vi "Report Creator.vi"(8 "date":string="total", 9 "Affiliate Weekly Path":path=path "C:/Dropbox/The_Student_Book_Project_LLC/Reports/affiliate.csv", 11 "Merch Weekly Path":path=path "C:/Dropbox/The_Student_Book_Project_LLC/Reports/Merchandise.csv") -> ()   [LabVIEW 2010]
uses:
  <vilib>/Utility/file.llb/Read From Spreadsheet File (string).vi
  <vilib>/Utility/file.llb/Write To Spreadsheet File (string).vi
  <vilib>/Analysis/NI_AALBase.lvlib
panel:
  out "Total Good Matches":string[][](array[string])
  out "Muliples Decided as Single":string[][](array[string])
  out "Levianthing 5":u8
  out "Levianthing 4":u8
  out "Levianthing 3":u8
  out "Levianthin 2":u8
  out "Affiliate Row # 5":i32
  out "Affiliate Row # 4":i32
  out "Affiliate Row # 3":i32
  out "Affiliate Row # 2":i32
  out "size(s)":i32
  out "Single Good Array":string[](array[string])
  out "Good Single Match Books per Org":string[][](array[string])
  out "Aggregated Good Multiple Match Books per Org":string[][](array[string])
  out "number of good, multiple matches":dbl
  out "Book Identifier":string
  out "Extension":string
  in  "Cutoff for Levianthing":u8=10
  out "Match Link 5":string
  out "Match Link 4":string
  out "Match Link 3":string
  out "Match Link 2":string
  out "Single Match Link":string
  out "Book Commission":string
  out "Book Revenue":string
  out "Book Name Merchandise":string
  out "Merchandise Data":string[][](array[string])
  out "Affiliate Row #":i32
  out "Merchandise row #":i32
  out "Single Match":bool
  out "Histogram Graph 2":T1(graph)
  out "number of good, single matches":dbl
  out "number not single and greater than 10":dbl
  out "number of bad matches":dbl
  out "number of good matches":dbl
  out "number of single matches":dbl
  out "number of multiple matches":dbl
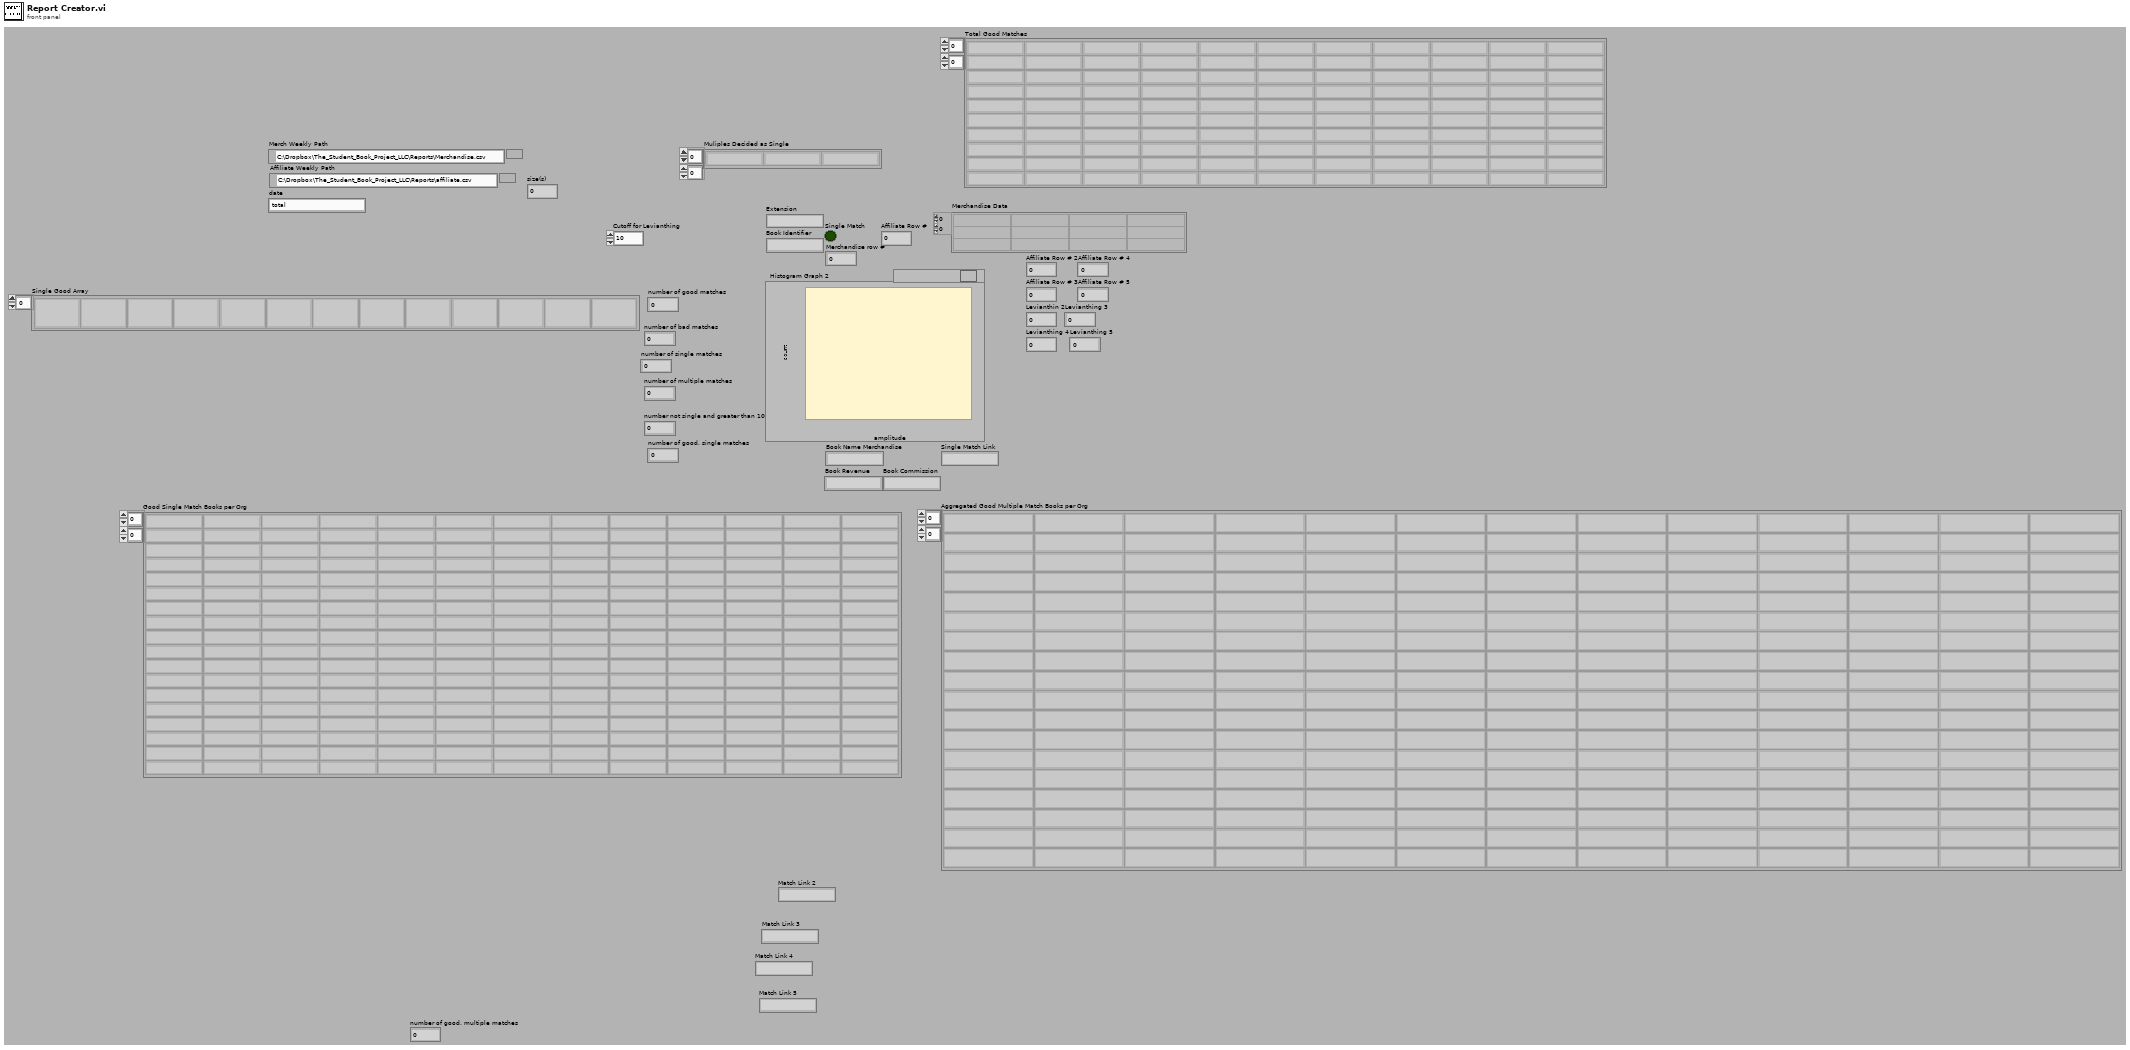
[diagram p1: front panel]
types:
  T1 = cluster{"X Values":dbl[], "Histogram: h(x)":i32[]}
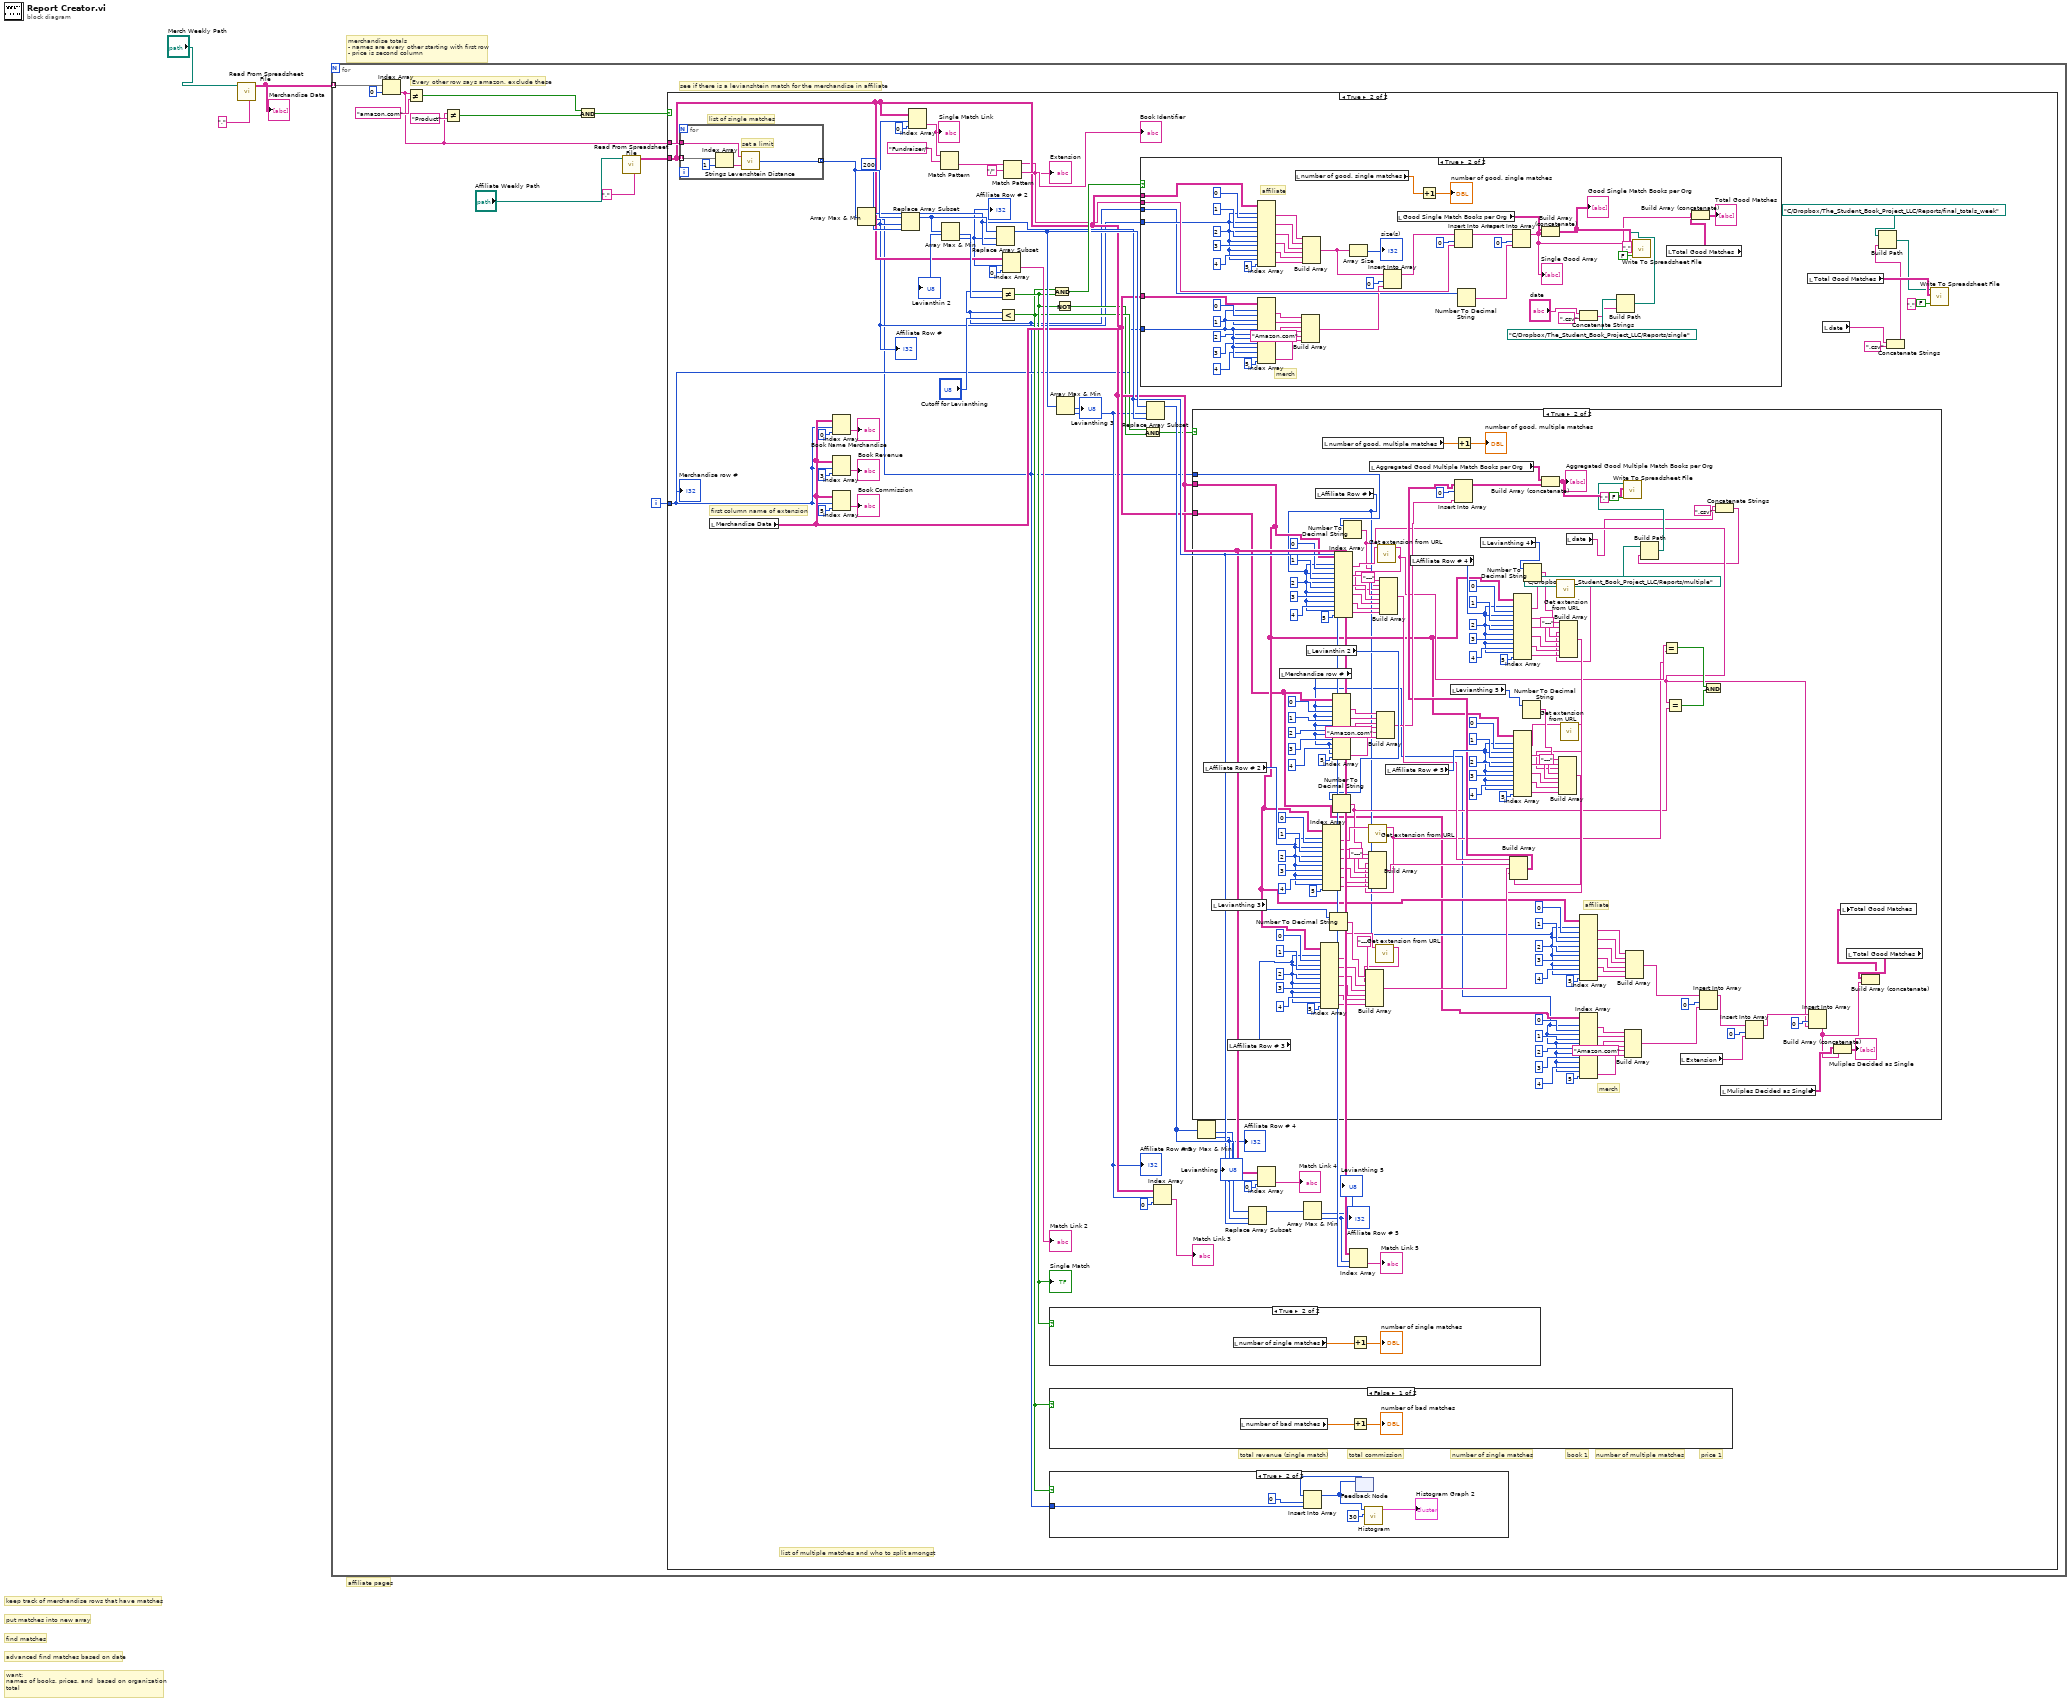
[diagram p0: block diagram]
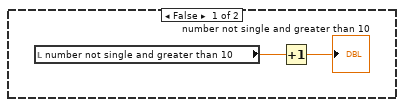
[diagram p5: hidden frame]
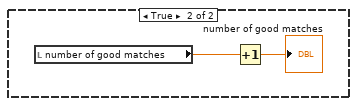
[diagram p6: hidden frame]
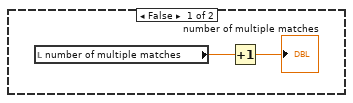
[diagram p7: hidden frame]
diagram:
  # "want:\nnames of books, prices, and  based on organization\ntotal"
  # "put matches into new array"
  # "keep track of merchandise rows that have matches"
  # "advanced find matches based on date"
  # "find matches"
  # "affiliate pages"
  # "merchandise totals\n- names are every other starting with first row\n- price is second column"
  n1 = call-poly <vilib>:"Read From Spreadsheet File.vi"("delimiter (\\t)"="," ("delimiter (\\t)"), "file path (dialog if empty)"="Merch Weekly Path") -> ("all rows"=w3:string[][])  [unwired: 5 in, 4 out]
  "Merchandise Data" <- w3
  n2 = for {
    tunnel: w3 -> [w10] mode=indexing
    i -> [w7]
    # "Every other row says amazon, exclude these"
    # "see if there is a levianshtein match for the merchandise in affiliate"
    n3 = Index Array(array=w10, index=0) -> (element=w9:string)
    n4 = Not Equal?(x=w9, y="amazon.com") -> (x != y?=w12:bool)
    n5 = Not Equal?(x=w9, y="Product") -> (x != y?=w11:bool)
    n6 = And(x=w12, y=w11) -> (x .and. y?=w5:bool)
    n7 = call-poly <vilib>:"Read From Spreadsheet File.vi"("delimiter (\\t)"="," ("delimiter (\\t)"), "file path (dialog if empty)"="Affiliate Weekly Path") -> ("all rows"=w6:string[][])  [unwired: 5 in, 4 out]
    n8 = case shown="True" w5 {
      tunnel: w9 -> [_ w69]
      tunnel: w6 -> [_ w39]
      tunnel: w7 -> [_ w33]
      frame False {
      }
      frame True {
        w46 = u8 200 ("new element/subarray")
        # "list of multiple matches and who to split amongst"
        # "list of single matches"
        # "total revenue (single match)"
        # "price 1"
        # "book 1"
        # "number of multiple matches"
        # "number of single matches"
        # "total commission"
        # "first column name of extension"
        n9 = for {
          tunnel: w69 -> [w302]
          tunnel: w39 -> [w301] mode=indexing
          tunnel: [w298] -> w68 mode=indexing
          # "set a limit"
          n10 = Index Array(array=w301, index=1) -> (element=w299:string)
          n11 = call "Strings Levenshtein Distance.vi"("String 2"=w299, "String 1"=w302) -> ("distance"=w298:u8)
        }
        n12 = local read "Merchandise Data"() -> (w40:string[][])
        n13 = Index Array(array=w40, index (row)=w33, index (col)=0 ("disabled index (col)")) -> (element=→"Book Name Merchandise":string)
        n14 = Index Array(array=w40, index (row)=w33, index (col)=3 ("disabled index (col)")) -> (element=→"Book Revenue":string)
        n15 = Index Array(array=w40, index (row)=w33, index (col)=5 ("disabled index (col)")) -> (element=→"Book Commission":string)
        n16 = Array Max & Min(array=w68) -> (min value=w27:u8, min index (indices)=w32:i32)  [unwired: 2 out]
        "Affiliate Row #" <- w32
        n17 = Replace Array Subset(array=w68, new element=w46, index=w32) -> (w66:u8[])
        n18 = Index Array(array=w39, index (row)=w32, index (col)=0 ("disabled index (col)")) -> (element=w45:string)
        "Single Match Link" <- w45
        n19 = Match Pattern(string=w45, regular expression="Fundraiser/") -> (after substring=w43:string)  [unwired: 1 in, 3 out]
        n20 = Array Max & Min(array=w66) -> (min value=w67:u8, min index (indices)=w31:i32)  [unwired: 2 out]
        "Affiliate Row # 2" <- w31
        "Levianthin 2" <- w67
        n21 = Replace Array Subset(array=w66, new element=w46, index=w31) -> (w49:u8[])
        n22 = Not Equal?(x=w27, y=w67) -> (x != y?=w38:bool)
        "Single Match" <- w38
        n23 = Less?(x=w27, y="Cutoff for Levianthing") -> (x < y?=w37:bool)
        n24 = Index Array(array=w39, index (row)=w31, index (col)=0 ("disabled index (col)")) -> (element=→"Match Link 2":string)
        n25 = Match Pattern(string=w43, regular expression="/") -> (before substring=w34:string, after substring=→"Book Identifier":string)  [unwired: 1 in, 2 out]
        "Extension" <- w34
        n26 = case shown="True" w38 {
          frame False {
            n27 = local read "number of multiple matches"() -> (w294:dbl)
            n28 = Increment(x=w294) -> (x+1=→"number of multiple matches":dbl)
          }
          frame True {
            n29 = local read "number of single matches"() -> (w296:dbl)
            n30 = Increment(x=w296) -> (x+1=→"number of single matches":dbl)
          }
        }
        n31 = case shown="False" w37 {
          frame False {
            n32 = local read "number of bad matches"() -> (w290:dbl)
            n33 = Increment(x=w290) -> (x+1=→"number of bad matches":dbl)
          }
          frame True {
            n34 = local read "number of good matches"() -> (w292:dbl)
            n35 = Increment(x=w292) -> (x+1=→"number of good matches":dbl)
          }
        }
        n36 = case shown="True" w37 {
          tunnel: w27 -> [_ w234]
          frame False {
          }
          frame True {
            n37 = feedback #1() -> (w230:u8[])  [unwired: 1 in]
            n38 = Insert Into Array(array=w230, index=0, new element=w234) -> (w229:u8[])
            n39 = feedback-in #1(w229) -> ()
            n40 = call <vilib>:"Histogram.vi"("intervals"=30, "X"=w229) -> ("Histogram Graph"=→"Histogram Graph 2":T1)  [unwired: 6 in, 3 out]
          }
        }
        n41 = And(x=w37, y=w38) -> (x .and. y?=w65:bool)
        n42 = Not(x=w38) -> (.not. x?=w36:bool)
        n43 = Array Max & Min(array=w49) -> (min value=→"Levianthing 3":u8, min index (indices)=w30:i32)  [unwired: 2 out]
        "Affiliate Row # 3" <- w30
        n44 = case shown="True" w65 {
          tunnel: w40 -> [_ w287]
          tunnel: w39 -> [_ w267]
          tunnel: w34 -> [_ w284]
          tunnel: w33 -> [_ w279]
          tunnel: w32 -> [_ w259]
          tunnel: w27 -> [_ w252]
          frame False {
            n45 = local read "number not single and greater than 10"() -> (w235:dbl)
            n46 = Increment(x=w235) -> (x+1=→"number not single and greater than 10":dbl)
          }
          frame True {
            # "merch"
            # "affiliate"
            n47 = Index Array(array=w267, index (row) #1=w259, index (col) #1=0 ("disabled index (col)"), index (row) #2=w259, index (col) #2=1 ("disabled index (col)"), index (row) #3=w259, index (col) #3=2 ("disabled index (col)"), index (row) #4=w259, index (col) #4=3 ("disabled index (col)"), index (row) #5=w259, index (col) #5=4 ("disabled index (col)"), index (row) #6=w259, index (col) #6=5 ("disabled index (col)")) -> (element #1=w266:string, element #2=w260:string, element #3=w258:string, element #4=w257:string, element #5=w256:string, element #6=w255:string)
            n48 = Index Array(array=w287, index (row) #1=w279, index (col) #1=0 ("disabled index (col)"), index (row) #2=w279, index (col) #2=1 ("disabled index (col)"), index (row) #3=w279, index (col) #3=2 ("disabled index (col)"), index (row) #4=w279, index (col) #4=3 ("disabled index (col)"), index (row) #5=w279, index (col) #5=4 ("disabled index (col)"), index (row) #6=w279, index (col) #6=5 ("disabled index (col)")) -> (element #1=w281:string, element #2=w264:string, element #3=w263:string, element #4=w262:string, element #6=w261:string)  [unwired: 1 out]
            n49 = local read "number of good, single matches"() -> (w288:dbl)
            n50 = Build Array(w281, w264, w263, w262, "Amazon.com" ("element"), w261) -> (w280:string[])
            n51 = Build Array(w266, w260, w258, w257, w256, w255) -> (w265:string[])
            n52 = Array Size(array=w265) -> (size(s)=→"size(s)":i32)
            n53 = Insert Into Array(array=w265, index=0, new element=w280) -> (w250:string[])
            n54 = local read "Good Single Match Books per Org"() -> (w254:string[][])
            n55 = Increment(x=w288) -> (x+1=→"number of good, single matches":dbl)
            n56 = Insert Into Array(array=w250, index=0, new element=w284) -> (w249:string[])
            n57 = Number To Decimal String(number=w252) -> (decimal integer string=w251:string)  [unwired: 1 in]
            n58 = Insert Into Array(array=w249, index=0, new element=w251) -> (w243:string[])
            "Single Good Array" <- w243
            n59 = Build Array (concatenate)(w254, w243) -> (w248:string[][])
            "Good Single Match Books per Org" <- w248
            n60 = Concatenate Strings("date", ".csv" ("string")) -> (w238:string)
            n61 = Build Path(base path=path "C:/Dropbox/The_Student_Book_Project_LLC/Reports/single" ("file path (dialog if empty)"), name or relative path=w238) -> (appended path=w244:path)
            n62 = call-poly <vilib>:"Write To Spreadsheet File.vi"("delimiter (\\t)"="," ("delimiter (\\t)"), "append to file? (new file:F)"=FALSE, "2D data"=w248, "file path (dialog if empty)"=w244) -> ()  [unwired: 4 in, 1 out]
            n63 = local read "Total Good Matches"() -> (w241:string[][])
            n64 = Build Array (concatenate)(w241, w243) -> (→"Total Good Matches":string[][])
          }
        }
        n65 = And(x=w37, y=w36) -> (x .and. y?=w35:bool)
        n66 = Replace Array Subset(array=w49, new element=w46, index=w30) -> (w48:u8[])
        n67 = Index Array(array=w39, index (row)=w30, index (col)=0 ("disabled index (col)")) -> (element=→"Match Link 3":string)
        n68 = case shown="True" w35 {
          tunnel: w40 -> [_ w90]
          tunnel: w39 -> [_ w92]
          tunnel: w27 -> [_ w202]
          frame False {
          }
          frame True {
            # "merch"
            # "affiliate"
            n69 = local read "Affiliate Row # 2"() -> (w149:i32)
            n70 = local read "Levianthing 3"() -> (w144:u8)
            n71 = local read "Affiliate Row # 3"() -> (w148:i32)
            n72 = local read "Merchandise row #"() -> (w89:i32)
            n73 = local read "Levianthin 2"() -> (w145:u8)
            n74 = local read "Affiliate Row #"() -> (w91:i32)
            n75 = Index Array(array=w92, index (row) #1=w148, index (col) #1=0 ("disabled index (col)"), index (row) #2=w148, index (col) #2=1 ("disabled index (col)"), index (row) #3=w148, index (col) #3=2 ("disabled index (col)"), index (row) #4=w148, index (col) #4=3 ("disabled index (col)"), index (row) #5=w148, index (col) #5=4 ("disabled index (col)"), index (row) #6=w148, index (col) #6=5 ("disabled index (col)")) -> (element #1=w132:string, element #2=w182:string, element #3=w181:string, element #4=w180:string, element #5=w179:string, element #6=w178:string)
            n76 = local read "number of good, multiple matches"() -> (w227:dbl)
            n77 = Index Array(array=w92, index (row) #1=w149, index (col) #1=0 ("disabled index (col)"), index (row) #2=w149, index (col) #2=1 ("disabled index (col)"), index (row) #3=w149, index (col) #3=2 ("disabled index (col)"), index (row) #4=w149, index (col) #4=3 ("disabled index (col)"), index (row) #5=w149, index (col) #5=4 ("disabled index (col)"), index (row) #6=w149, index (col) #6=5 ("disabled index (col)")) -> (element #1=w133:string, element #2=w194:string, element #3=w193:string, element #4=w192:string, element #5=w191:string, element #6=w190:string)
            n78 = Number To Decimal String(number=w144) -> (decimal integer string=w177:string)  [unwired: 1 in]
            n79 = Index Array(array=w90, index (row) #1=w89, index (col) #1=0 ("disabled index (col)"), index (row) #2=w89, index (col) #2=1 ("disabled index (col)"), index (row) #3=w89, index (col) #3=2 ("disabled index (col)"), index (row) #4=w89, index (col) #4=3 ("disabled index (col)"), index (row) #5=w89, index (col) #5=4 ("disabled index (col)"), index (row) #6=w89, index (col) #6=5 ("disabled index (col)")) -> (element #1=w212:string, element #2=w206:string, element #3=w205:string, element #4=w204:string, element #6=w203:string)  [unwired: 1 out]
            n80 = Number To Decimal String(number=w145) -> (decimal integer string=w118:string)  [unwired: 1 in]
            n81 = Index Array(array=w92, index (row) #1=w91, index (col) #1=0 ("disabled index (col)"), index (row) #2=w91, index (col) #2=1 ("disabled index (col)"), index (row) #3=w91, index (col) #3=2 ("disabled index (col)"), index (row) #4=w91, index (col) #4=3 ("disabled index (col)"), index (row) #5=w91, index (col) #5=4 ("disabled index (col)"), index (row) #6=w91, index (col) #6=5 ("disabled index (col)")) -> (element #1=w134:string, element #2=w218:string, element #3=w217:string, element #4=w216:string, element #5=w215:string, element #6=w214:string)
            n82 = Number To Decimal String(number=w202) -> (decimal integer string=w80:string)  [unwired: 1 in]
            n83 = call "Get extension from URL.vi"("url"=w133) -> ("Extension"=w119:string)  [unwired: 10 in]
            n84 = Build Array("---" ("element"), w118, w119, w194, w193, w192, w191, w190) -> (w140:string[])
            n85 = local read "Aggregated Good Multiple Match Books per Org"() -> (w225:string[][])
            n86 = call "Get extension from URL.vi"("url"=w132) -> ("Extension"=w131:string)  [unwired: 10 in]
            n87 = Build Array("---" ("element"), w177, w131, w182, w181, w180, w179, w178) -> (w139:string[])
            n88 = Build Array(w212, w206, w205, w204, "Amazon.com" ("element"), w203) -> (w136:string[])
            n89 = call "Get extension from URL.vi"("url"=w134) -> ("Extension"=w120:string)  [unwired: 10 in]
            n90 = Build Array("---" ("element"), w80, w120, w218, w217, w216, w215, w214) -> (w141:string[])
            n91 = local read "Affiliate Row # 5"() -> (w146:i32)
            n92 = local read "Affiliate Row # 4"() -> (w147:i32)
            n93 = local read "Levianthing 5"() -> (w142:u8)
            n94 = Increment(x=w227) -> (x+1=→"number of good, multiple matches":dbl)
            n95 = local read "Levianthing 4"() -> (w143:u8)
            n96 = Index Array(array=w92, index (row) #1=w146, index (col) #1=0 ("disabled index (col)"), index (row) #2=w146, index (col) #2=1 ("disabled index (col)"), index (row) #3=w146, index (col) #3=2 ("disabled index (col)"), index (row) #4=w146, index (col) #4=3 ("disabled index (col)"), index (row) #5=w146, index (col) #5=4 ("disabled index (col)"), index (row) #6=w146, index (col) #6=5 ("disabled index (col)")) -> (element #1=w128:string, element #2=w156:string, element #3=w155:string, element #4=w154:string, element #5=w153:string, element #6=w152:string)
            n97 = Index Array(array=w92, index (row) #1=w147, index (col) #1=0 ("disabled index (col)"), index (row) #2=w147, index (col) #2=1 ("disabled index (col)"), index (row) #3=w147, index (col) #3=2 ("disabled index (col)"), index (row) #4=w147, index (col) #4=3 ("disabled index (col)"), index (row) #5=w147, index (col) #5=4 ("disabled index (col)"), index (row) #6=w147, index (col) #6=5 ("disabled index (col)")) -> (element #1=w130:string, element #2=w169:string, element #3=w168:string, element #4=w167:string, element #5=w166:string, element #6=w165:string)
            n98 = Number To Decimal String(number=w142) -> (decimal integer string=w151:string)  [unwired: 1 in]
            n99 = Number To Decimal String(number=w143) -> (decimal integer string=w164:string)  [unwired: 1 in]
            n100 = call "Get extension from URL.vi"("url"=w130) -> ("Extension"=w129:string)  [unwired: 10 in]
            n101 = Build Array("---" ("element"), w164, w129, w169, w168, w167, w166, w165) -> (w138:string[])
            n102 = call "Get extension from URL.vi"("url"=w128) -> ("Extension"=w127:string)  [unwired: 10 in]
            n103 = Build Array("---" ("element"), w151, w127, w156, w155, w154, w153, w152) -> (w137:string[])
            n104 = Build Array(w141, w140, w139, w138, w137) -> (w135:string[][])
            n105 = Insert Into Array(array=w135, index (row)=0 ("index"), new element=w136) -> (w126:string[][])  [unwired: 1 in]
            n106 = Build Array (concatenate)(w225, w126) -> (w125:string[][])
            "Aggregated Good Multiple Match Books per Org" <- w125
            n107 = local read "date"() -> (w73:string)
            n108 = Index Array(array=w92, index (row) #1=w91, index (col) #1=0 ("disabled index (col)"), index (row) #2=w91, index (col) #2=1 ("disabled index (col)"), index (row) #3=w91, index (col) #3=2 ("disabled index (col)"), index (row) #4=w91, index (col) #4=3 ("disabled index (col)"), index (row) #5=w91, index (col) #5=4 ("disabled index (col)"), index (row) #6=w91, index (col) #6=5 ("disabled index (col)")) -> (element #1=w102:string, element #2=w97:string, element #3=w96:string, element #4=w95:string, element #5=w94:string, element #6=w93:string)
            n109 = Index Array(array=w90, index (row) #1=w89, index (col) #1=0 ("disabled index (col)"), index (row) #2=w89, index (col) #2=1 ("disabled index (col)"), index (row) #3=w89, index (col) #3=2 ("disabled index (col)"), index (row) #4=w89, index (col) #4=3 ("disabled index (col)"), index (row) #5=w89, index (col) #5=4 ("disabled index (col)"), index (row) #6=w89, index (col) #6=5 ("disabled index (col)")) -> (element #1=w114:string, element #2=w101:string, element #3=w100:string, element #4=w99:string, element #6=w98:string)  [unwired: 1 out]
            n110 = Build Array(w114, w101, w100, w99, "Amazon.com" ("element"), w98) -> (w86:string[])
            n111 = Build Array(w102, w97, w96, w95, w94, w93) -> (w87:string[])
            n112 = Equal?(x=w120, y=w119) -> (x = y?=w117:bool)
            n113 = Equal?(x=w80, y=w118) -> (x = y?=w116:bool)
            n114 = local read "Extension"() -> (w81:string)
            n115 = Insert Into Array(array=w87, index=0, new element=w86) -> (w84:string[])
            n116 = And(x=w117, y=w116) -> ()  [unwired: 1 out]
            n117 = Concatenate Strings(w73, ".csv" ("string")) -> (w72:string)
            n118 = Build Path(base path=path "C:/Dropbox/The_Student_Book_Project_LLC/Reports/multiple" ("file path (dialog if empty)"), name or relative path=w72) -> (appended path=w121:path)
            n119 = call-poly <vilib>:"Write To Spreadsheet File.vi"("delimiter (\\t)"="," ("delimiter (\\t)"), "append to file? (new file:F)"=FALSE, "2D data"=w125, "file path (dialog if empty)"=w121) -> ()  [unwired: 4 in, 1 out]
            n120 = local read "Muliples Decided as Single"() -> (w78:string[][])
            n121 = Insert Into Array(array=w84, index=0, new element=w81) -> (w82:string[])
            n122 = Insert Into Array(array=w82, index=0, new element=w80) -> (w77:string[])
            n123 = Build Array (concatenate)(w78, w77) -> (→"Muliples Decided as Single":string[][])
            n124 = local read "Total Good Matches"() -> (w76:string[][])
            n125 = Build Array (concatenate)(w76, w77) -> (w75:string[][])
            n126 = local write "Total Good Matches"(w75) -> ()
          }
        }
        n127 = Array Max & Min(array=w48) -> (min value=→"Levianthing 4":u8, min index (indices)=w29:i32)  [unwired: 2 out]
        "Affiliate Row # 4" <- w29
        n128 = Replace Array Subset(array=w48, new element=w46, index=w29) -> (w50:u8[])
        n129 = Index Array(array=w39, index (row)=w29, index (col)=0 ("disabled index (col)")) -> (element=→"Match Link 4":string)
        n130 = Array Max & Min(array=w50) -> (min value=→"Levianthing 5":u8, min index (indices)=w28:i32)  [unwired: 2 out]
        "Affiliate Row # 5" <- w28
        n131 = Index Array(array=w39, index (row)=w28, index (col)=w46) -> (element=→"Match Link 5":string)
        n132 = local read "Total Good Matches"() -> (w21:string[][])
        n133 = local read "date"() -> (w17:string)
        n134 = Concatenate Strings(w17, ".csv" ("string")) -> (w16:string)
        n135 = Build Path(base path=path "C:/Dropbox/The_Student_Book_Project_LLC/Reports/final_totals_week" ("file path (dialog if empty)"), name or relative path=w16) -> (appended path=w19:path)
        n136 = call-poly <vilib>:"Write To Spreadsheet File.vi"("delimiter (\\t)"="," ("delimiter (\\t)"), "append to file? (new file:F)"=FALSE, "2D data"=w21, "file path (dialog if empty)"=w19) -> ()  [unwired: 4 in, 1 out]
        "Merchandise row #" <- w33
      }
    }
  }
